vi "Timestamp with Date and Time Strings.vi"(9 "Delimiter (Time)":string="_", 10 "Delimiter (Date)":string="_", 11 "Timestamp Format String":string="%Y%m%d_%H%M%S") -> (1 "Time String":string="10_48_09 AM", 2 "Date String":string="2_5_2020", 3 "Timestamp String":string="20200205_104809")   [LabVIEW 2015]
panel:
  in  "Date Format":enum16{"short", "long", "abbreviated"}(ring)
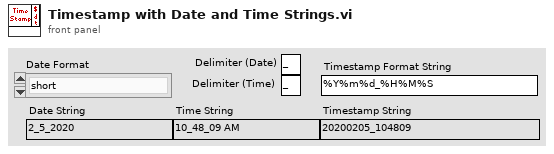
[diagram p1: front panel]
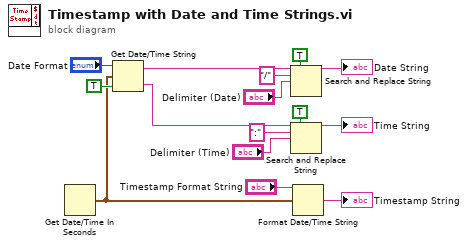
[diagram p0: block diagram]
diagram:
  n1 = Get Date/Time In Seconds() -> (seconds since 1Jan1904=w2:timestamp)
  n2 = Get Date/Time String(date format (0)="Date Format", seconds (now)=w2, want seconds? (F)=TRUE) -> (date string=w13:string, time string=w6:string)
  n3 = Search and Replace String(replace all?=TRUE ("replace all? (F)"), input string=w13, search string="/", replace string="Delimiter (Date)") -> (result string=→"Date String":string)  [unwired: 4 in, 3 out]
  n4 = Search and Replace String(replace all?=TRUE ("replace all? (F)"), input string=w6, search string=":", replace string="Delimiter (Time)") -> (result string=→"Time String":string)  [unwired: 4 in, 3 out]
  n5 = Format Date/Time String(time format string (%c)="Timestamp Format String", seconds (now)=w2) -> (date/time string=→"Timestamp String":string)  [unwired: 1 in]
